vi "Decimal Value.vi"(7 "Type":string, 10 "Decimal":u16, 11 "Data In":string) -> (3 "Data Out":string)   [LabVIEW 2020]
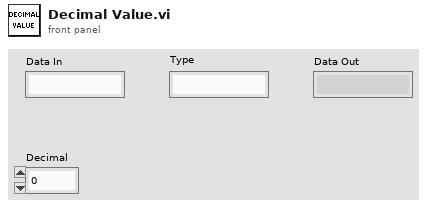
[diagram p1: front panel]
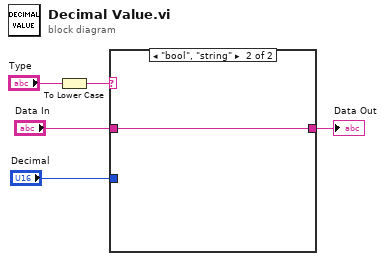
[diagram p0: block diagram]
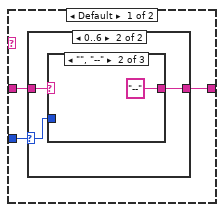
[diagram p2: hidden frame]
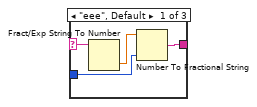
[diagram p4: hidden frame]
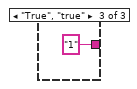
[diagram p5: hidden frame]
diagram:
  n1 = To Lower Case(string="Type") -> (all lower case string=w1:string)
  n2 = case shown="\"bool\", \"string\"" w1 {
    tunnel: "Decimal" -> [w8 _]
    tunnel: "Data In" -> [w7 w19]
    tunnel: [w6 w19] -> w3
    frame Default {
      n3 = case shown="0..6" w8 {
        selector: w8 -> [_ w11]
        tunnel: w7 -> [w9 w12]
        tunnel: [w9 w10] -> w6
        frame 999, Default {
        }
        frame 0..6 {
          n4 = case shown="\"\", \"--\"" w12 {
            selector: w12 -> [w16 _ _]
            tunnel: w11 -> [w14 _ _]
            tunnel: [w13 "--" "1"] -> w10
            frame "eee", Default {
              n5 = Fract/Exp String To Number(string=w16) -> (number=w15:dbl)  [unwired: 3 in, 1 out]
              n6 = Number To Fractional String(number=w15, precision (6)=w14) -> (F-format string=w13:string)  [unwired: 2 in]
            }
            frame "", "--" {
            }
            frame "True", "true" {
            }
          }
        }
      }
    }
    frame "bool", "string" {
    }
  }
  "Data Out" <- w3
